vi "NPL Joerger Sample Time Calc.vi"(9 "# Samples":u32=2000 min=1 max=262143 step=1, 11 "Acquisition Rate":u16(ring) items=["40 MHz", "20 MHz", "10 MHz", "5 MHz", "2.5 MHz", "1 MHz", "100 kHz", "10 kHz"]) -> (3 "Sample Time":dbl caption="s" format="%^#_3g")   [LabVIEW 2013]
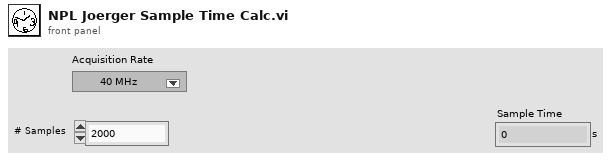
[diagram p1: front panel]
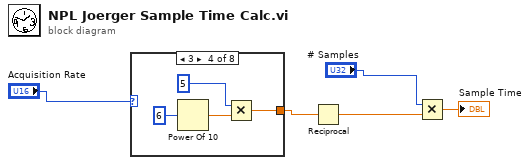
[diagram p0: block diagram]
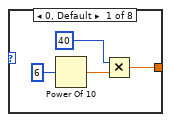
[diagram p2: hidden frame]
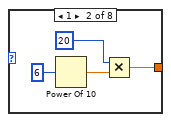
[diagram p3: hidden frame]
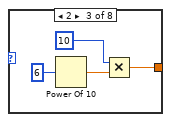
[diagram p4: hidden frame]
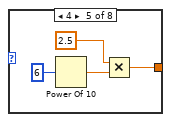
[diagram p5: hidden frame]
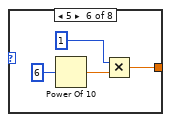
[diagram p6: hidden frame]
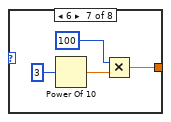
[diagram p7: hidden frame]
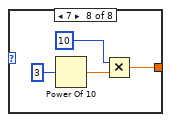
[diagram p8: hidden frame]
diagram:
  n1 = case shown="3" "Acquisition Rate" {
    tunnel: [w6 w10 w14 w18 w22 w26 w30 w34] -> w3
    frame 0, Default {
      n2 = Power Of 10(x=6) -> (10^x=w8:dbl)
      n3 = Multiply(x=40, y=w8) -> (x*y=w6:dbl)
    }
    frame 1 {
      n4 = Power Of 10(x=6) -> (10^x=w12:dbl)
      n5 = Multiply(x=20, y=w12) -> (x*y=w10:dbl)
    }
    frame 2 {
      n6 = Power Of 10(x=6) -> (10^x=w16:dbl)
      n7 = Multiply(x=10, y=w16) -> (x*y=w14:dbl)
    }
    frame 3 {
      n8 = Power Of 10(x=6) -> (10^x=w20:dbl)
      n9 = Multiply(x=5, y=w20) -> (x*y=w18:dbl)
    }
    frame 4 {
      n10 = Power Of 10(x=6) -> (10^x=w24:dbl)
      n11 = Multiply(x=2.5, y=w24) -> (x*y=w22:dbl)
    }
    frame 5 {
      n12 = Power Of 10(x=6) -> (10^x=w28:dbl)
      n13 = Multiply(x=1, y=w28) -> (x*y=w26:dbl)
    }
    frame 6 {
      n14 = Power Of 10(x=3) -> (10^x=w32:dbl)
      n15 = Multiply(x=100, y=w32) -> (x*y=w30:dbl)
    }
    frame 7 {
      n16 = Power Of 10(x=3) -> (10^x=w36:dbl)
      n17 = Multiply(x=10, y=w36) -> (x*y=w34:dbl)
    }
  }
  n18 = Reciprocal(x=w3) -> (1/x=w4:dbl)
  n19 = Multiply(x="# Samples", y=w4) -> (x*y=→"Sample Time":dbl)
